vi "Main.vi"(8 "error in (no error)":errorcluster, 10 "ControllerQ":refnum<queue>) -> (0 "error out":errorcluster, 3 "ModuleQ Out":refnum<queue>)   [LabVIEW 2020, in "ErrorHandler.lvlib"]
doc: "Use this template to build a producer/consumer design pattern with events to produce queue items. Use this design pattern instead of the User Interface Event Handler pattern for user interfaces when you want to execute code asynchronously in response to an event without slowing the user interface responsiveness."
uses:
  ErrorHandler.lvlib
  Controller/Controls/QMessage.ctl
  Controls/QMessage.ctl
  Controls/ConsummerLoopData.ctl
  Controls/EventLoopData.ctl
  Controller/Controller.lvlib
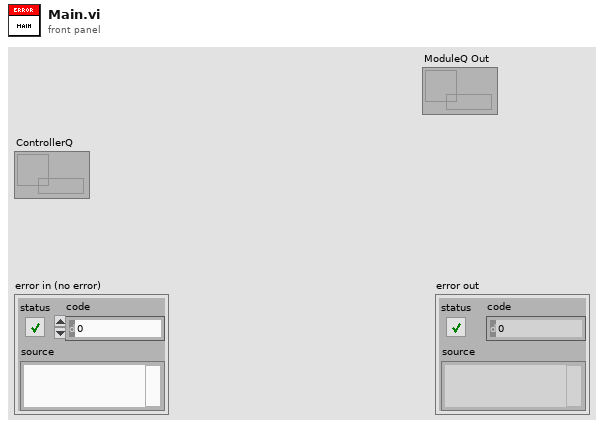
[diagram p1: front panel]
types:
  T1 = typedef "ErrorHandler.lvlib/EventLoopData.ctl" = cluster{"DummyData":dbl}
  T2 = typedef "ErrorHandler.lvlib/ConsummerLoopData.ctl" = cluster{"Error File Refnum":refnum<file>}
  T3 = typedef "Controller.lvlib/QMessage.ctl" = cluster{"Message":string, "Data":variant}
  T4 = typedef "ErrorHandler.lvlib/QMessage.ctl" = cluster{"Message":string, "Data":errorcluster}
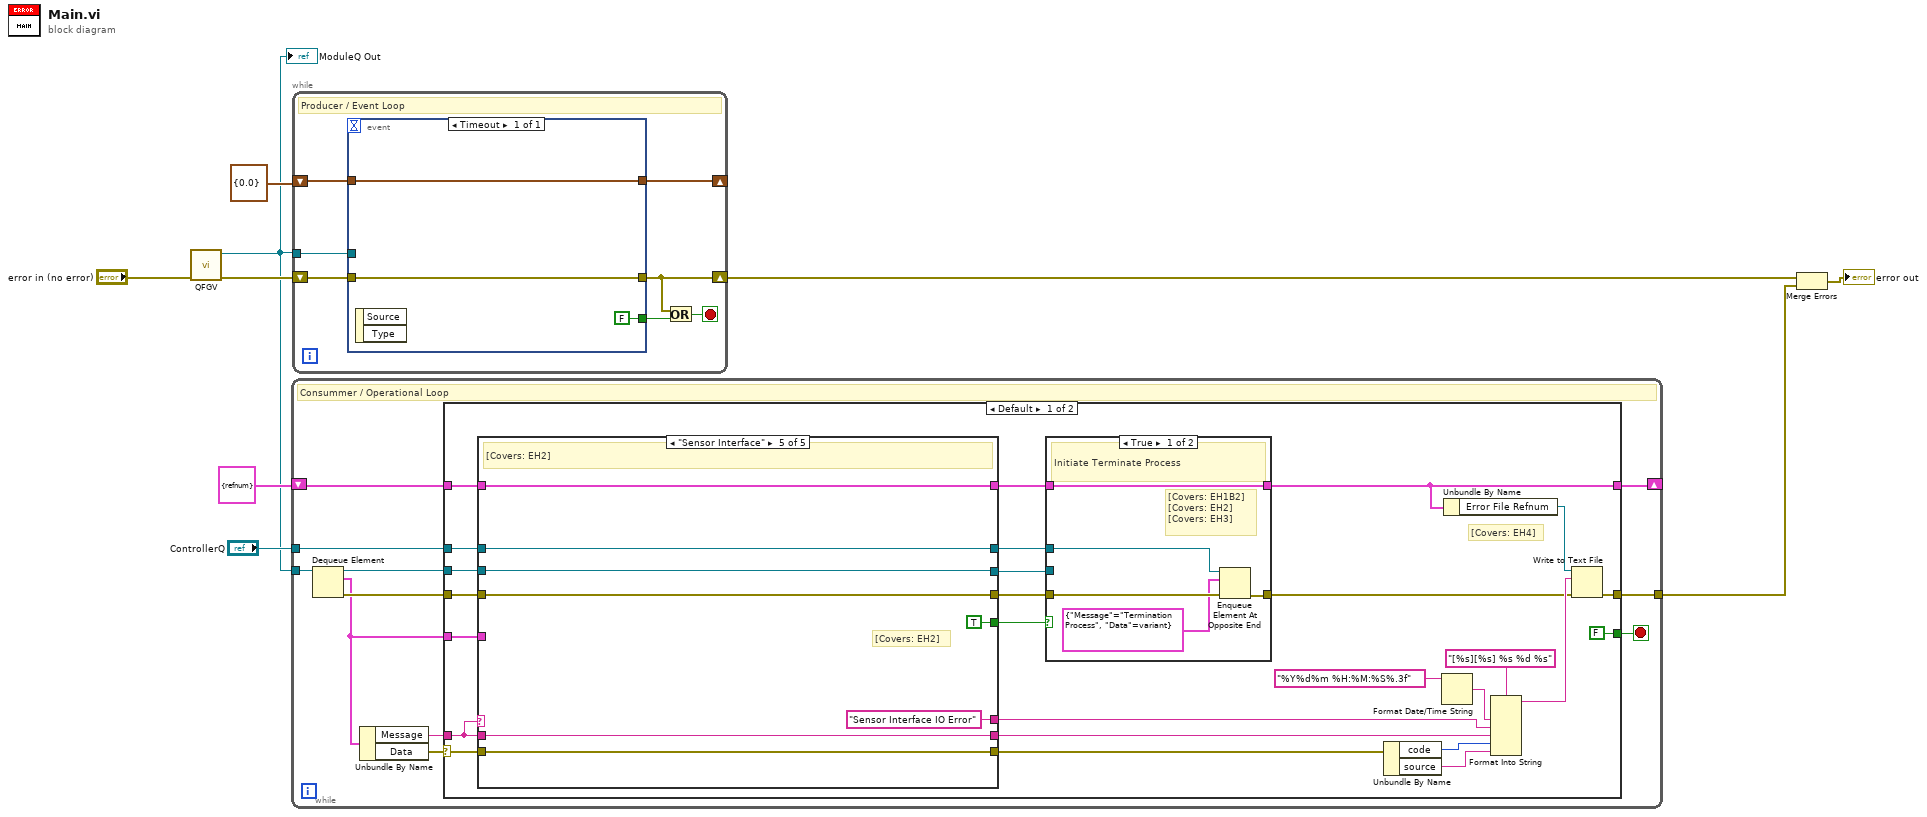
[diagram p0: block diagram]
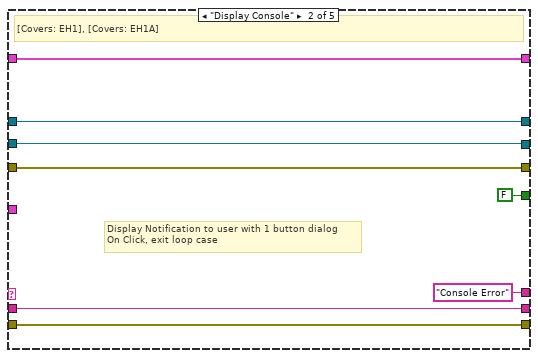
[diagram p4: hidden frame]
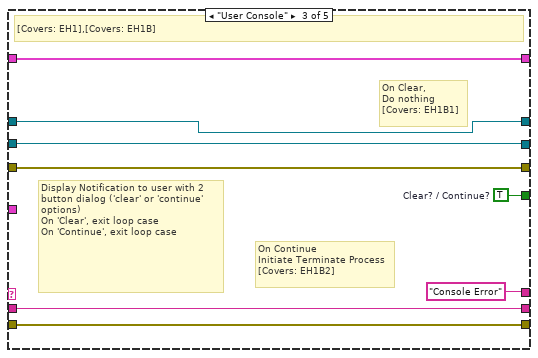
[diagram p5: hidden frame]
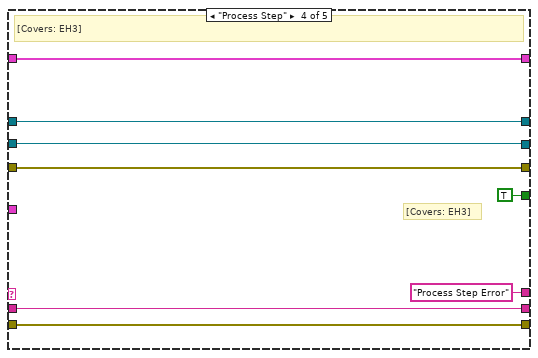
[diagram p6: hidden frame]
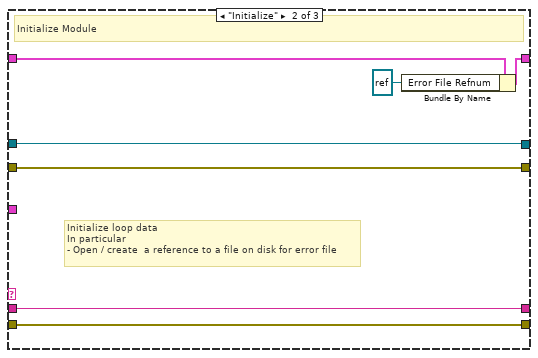
[diagram p8: hidden frame]
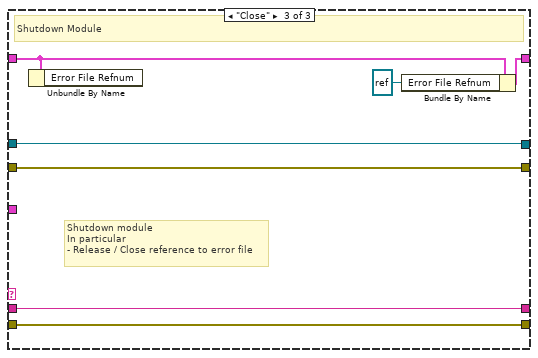
[diagram p9: hidden frame]
diagram:
  n1 = call "QFGV.vi"("error in (no error)"="error in (no error)") -> ("error out"=w2:errorcluster, "ModuleQ"=w1:refnum<queue>)  [unwired: 9 in]
  "ModuleQ Out" <- w1
  n2 = while {
    tunnel: w1 -> [w20]
    shift-right: [w18] -> _
    shift-left: T2 {"Error File Refnum"=refnum} -> [w17]
    tunnel: [w15] -> w8
    tunnel: "ControllerQ" -> [w10]
    stop <- w19 stop-if-true
    # "Consummer / Operational Loop"
    n3 = Dequeue Element(queue=w20) -> (queue out=w12:refnum<queue>, element=w11:T4, error out=w16:errorcluster)  [unwired: 2 in, 1 out]
    n4 = Unbundle By Name(w11) -> ("Message"=w13:string, "Data"=w14:errorcluster)
    n5 = case shown="Default" w14 {
      selector: w14 -> [w42 w94]
      tunnel: [FALSE _] -> w19
      tunnel: [w28 w96] -> w18
      tunnel: w17 -> [w44 w98]
      tunnel: w16 -> [w45 w99]
      tunnel: [w40 w95] -> w15
      tunnel: w13 -> [w37 w93]
      tunnel: w12 -> [w43 w97]
      tunnel: w11 -> [w41 w92]
      tunnel: w10 -> [w22 _]
      frame Default {
        # "[Covers: EH4]"
        n6 = case shown="\"Sensor Interface\"" w37 {
          tunnel: [w59 w67 w74 w82 w90] -> w26
          tunnel: w45 -> [w59 w67 w74 w82 w90]
          tunnel: [w58 w66 w75 w83 w91] -> w29
          tunnel: w44 -> [w58 w66 w75 w83 w91]
          tunnel: w43 -> [w55 w63 w73 w81 w89]
          tunnel: w42 -> [w57 w65 w72 w80 w88]
          tunnel: w41 -> [_ _ _ _ _]
          tunnel: [w57 w65 w72 w80 w88] -> w36
          tunnel: [w56 w64 w71 w79 w87] -> w35
          tunnel: w37 -> [w56 w64 w71 w79 w87]
          tunnel: [_ "Console Error" ("Message") "Console Error" ("Message") "Process Step Error" ("Message") "Sensor Interface IO Error" ("Message")] -> w24
          tunnel: [w55 w63 w73 w81 w89] -> w27
          tunnel: [_ FALSE ("Clear? / Continue?") w70 TRUE ("Clear? / Continue?") TRUE ("Clear? / Continue?")] -> w23
          tunnel: w22 -> [w54 w60 w68 w76 w84]
          tunnel: [w54 w60 w68 w76 w84] -> w21
          frame Default {
          }
          frame "Display Console" {
            # "Display Notification to user with 1 button dialog\nOn Click, exit loop case"
            # "[Covers: EH1], [Covers: EH1A]"
          }
          frame "User Console" {
            w70 = TRUE  # Clear? / Continue?
            # "On Continue\nInitiate Terminate Process\n[Covers: EH1B2]"
            # "On Clear,\nDo nothing\n[Covers: EH1B1]"
            # "Display Notification to user with 2 button dialog ('clear' or 'continue' options)\nOn 'Clear', exit loop case\nOn 'Continue', exit loop case"
            # "[Covers: EH1],[Covers: EH1B]"
          }
          frame "Process Step" {
            # "[Covers: EH3]"
            # "[Covers: EH3]"
          }
          frame "Sensor Interface" {
            # "[Covers: EH2]"
            # "[Covers: EH2]"
          }
        }
        n7 = case shown="True" w23 {
          tunnel: [w49 w53] -> w25
          tunnel: w26 -> [w50 w53]
          tunnel: [w51 w52] -> w28
          tunnel: w29 -> [w51 w52]
          tunnel: w27 -> [_ _]
          tunnel: w21 -> [w48 _]
          frame True {
            # "[Covers: EH1B2] \n[Covers: EH2] \n[Covers: EH3]"
            # "Initiate Terminate Process"
            n8 = Enqueue Element At Opposite End(queue=w48, element=T3 {"Message"="Termination Process", "Data"=variant}, error in (no error)=w50) -> (error out=w49:errorcluster)  [unwired: 1 in, 2 out]
          }
          frame False {
          }
        }
        n9 = Unbundle By Name(w36) -> ("code"=w33:i32, "source"=w32:string)
        n10 = Format Date/Time String(time format string (%c)="%Y%d%m %H:%M:%S%.3f") -> (date/time string=w30:string)  [unwired: 2 in]
        n11 = Unbundle By Name(w28) -> ("Error File Refnum"=w39:refnum<file>)
        n12 = Format Into String(format string="[%s][%s] %s %d %s", w30, w24, w35, w33, w32) -> (resulting string=w38:string)  [unwired: 2 in, 1 out]
        n13 = Write to Text File(file (use dialog)=w39, text=w38, error in=w25) -> (error out=w40:errorcluster)  [unwired: 1 in, 2 out]
      }
      frame No Error {
        n14 = case shown="Default" w93 {
          tunnel: [w104 w111 w118] -> w95
          tunnel: w99 -> [w104 w111 w118]
          tunnel: [w103 w106 w114] -> w96
          tunnel: w98 -> [w103 w107 w112]
          tunnel: w97 -> [w100 w108 w115]
          tunnel: w94 -> [w102 w110 w117]
          tunnel: [w102 w110 w117] -> _
          tunnel: [w101 w109 w116] -> _
          tunnel: w93 -> [w101 w109 w116]
          tunnel: [w100 w108 w115] -> _
          tunnel: w92 -> [_ _ _]
          frame Default {
          }
          frame "Initialize" {
            # "Initialize loop data\nIn particular\n- Open / create  a reference to a file on disk for error file"
            # "Initialize Module"
            n15 = Bundle By Name(cluster=w107, "Error File Refnum"=refnum<file> refnum) -> (w106:T2)
          }
          frame "Close" {
            # "Shutdown module\nIn particular\n- Release / Close reference to error file"
            # "Shutdown Module"
            n16 = Unbundle By Name(w112) -> ()  [unwired: 1 out]
            n17 = Bundle By Name(cluster=w112, "Error File Refnum"=refnum<file> refnum) -> (w114:T2)
          }
        }
      }
    }
  }
  n18 = while {
    shift-right: [w121] -> w7
    shift-left: w2 -> [w124]
    tunnel: w1 -> [w125]
    shift-right: [w120] -> _
    shift-left: T1 {"DummyData"=0.0} -> [w119]
    stop <- w122 stop-if-true
    # "Producer / Event Loop"
    n19 = event shown="[0] Timeout" {
      selector: _ -> [_]
      dyn-events: _ -> [_]
      timeout: _ -> [_]
      tunnel: w125 -> [_]
      tunnel: w124 -> [w127]
      tunnel: [w127] -> w121
      tunnel: [FALSE ("stop")] -> w123
      tunnel: [w128] -> w120
      tunnel: w119 -> [w128]
      event Timeout {
        n20 = event-data() -> ()  [unwired: 1 in, 2 out]
      }
    }
    n21 = Or(x=w121, y=w123) -> (x .or. y?=w122:bool)
  }
  n22 = Merge Errors(w7, w8) -> (→"error out":errorcluster)
